vi "Get Value Test.vi"(8 "error in (no error)":errorcluster caption="entrée d'erreur (pas d'erreur)", 11 "Class Camera  IV3-500CA - Read version en entrée":refnum<class "Class Camera  IV3-500CA - Read version.lvclass">) -> (0 "error out":errorcluster caption="sortie d'erreur", 2 "Value Test":string, 3 "Class Camera  IV3-500CA - Read version en sortie":refnum<class "Class Camera  IV3-500CA - Read version.lvclass">)   [LabVIEW 2020, in "Library Instrument & Equipement.lvlib" / "Library Camera.lvlib" / "Class Camera  IV3-500CA - Read version.lvclass"]
uses:
  Class Camera  IV3-500CA - Read version.lvclass
  Class Camera  IV3-500CA - Read version.lvclass/Class Camera  IV3-500CA - Read version.ctl
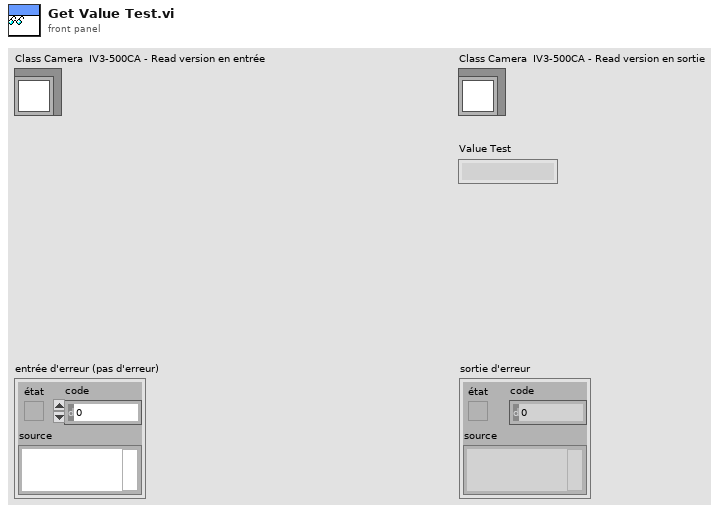
[diagram p1: front panel]
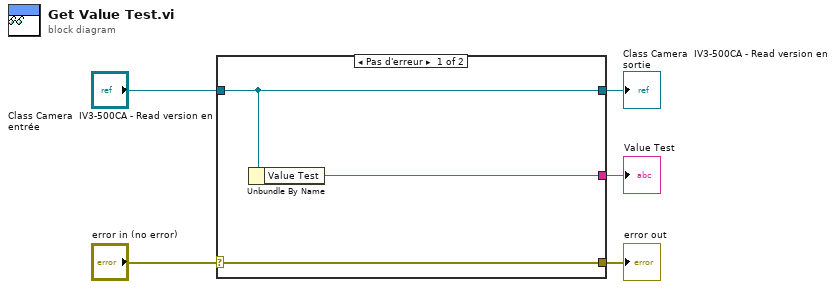
[diagram p0: block diagram]
diagram:
  n1 = case shown="Pas d'erreur" "error in (no error)" {
    selector: "error in (no error)" -> [w8 w9]
    tunnel: [w8 w9] -> w4
    tunnel: [w7 w10] -> w2
    tunnel: "Class Camera  IV3-500CA - Read version en entrée" -> [w7 w10]
    tunnel: [w6 _] -> w1
    frame No Error {
      n2 = Unbundle By Name(w7) -> ("Value Test"=w6:string)
    }
    frame Error {
    }
  }
  "error out" <- w4
  "Class Camera  IV3-500CA - Read version en sortie" <- w2
  "Value Test" <- w1
